vi "CD System Explorer lvlib.vi"(9 "Action":T1) -> (1 "Output":string)   [LabVIEW 2015, in "NIVS_Consolidated_CDW_MetaDataObj.lvclass"]
doc: "Constants, which are necessary for the <B>CD System Explorer library</B> in the generated custom device project."
uses:
  NIVS_Consolidated_CDW_MetaDataObj.lvclass
  CD System Explorer lvlib.ctl
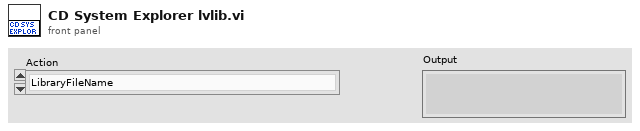
[diagram p1: front panel]
types:
  T1 = typedef "NIVS_Consolidated_CDW_MetaDataObj.lvclass/CD System Explorer lvlib.ctl" = enum16{"LibraryFileName", "LibraryFolderName", "System Explorer.FolderName", "System Explorer.Dynamically Called.FolderName", "System Explorer.Dynamically Called.Extra Pages.FolderName", "System Explorer.Dynamically Called.Extra Pages.TemplatePathAndName", "System Explorer.Dynamically Called.Main Page.VIName", "System Explorer.Dynamically Called.Main Page.TemplatePathAndName", "System Explorer.Dynamically Called.Initialization VI.VIName", "System Explorer.Dynamically Called.Initialization VI.TemplatePathAndName", "System Explorer.SubVI.FolderName", "System Explorer.Types.FolderName", "System Explorer.ActionVIOnCompile.VIName", "System Explorer.ExportConfigRTM.VIName", "System Explorer.LoadHelpFile.VIName"}
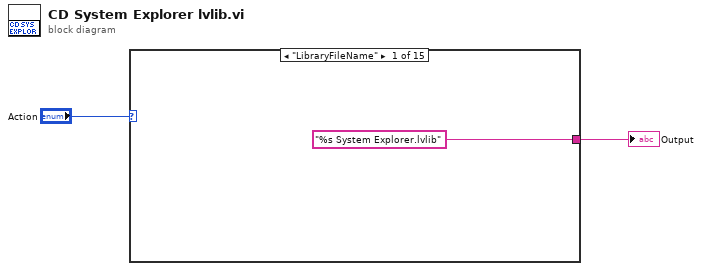
[diagram p0: block diagram]
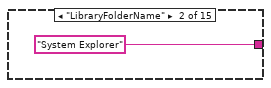
[diagram p2: hidden frame]
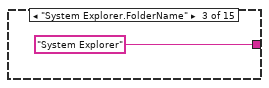
[diagram p3: hidden frame]
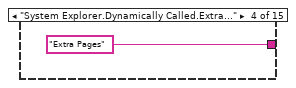
[diagram p4: hidden frame]
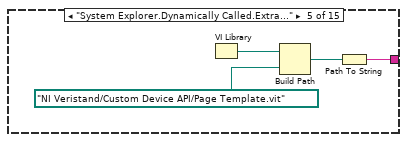
[diagram p5: hidden frame]
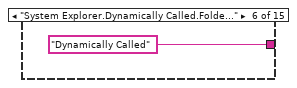
[diagram p6: hidden frame]
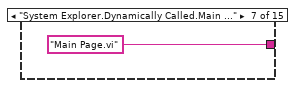
[diagram p7: hidden frame]
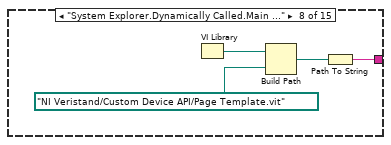
[diagram p8: hidden frame]
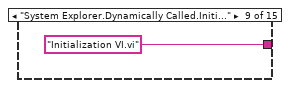
[diagram p9: hidden frame]
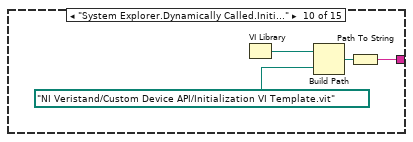
[diagram p10: hidden frame]
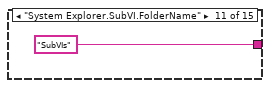
[diagram p11: hidden frame]
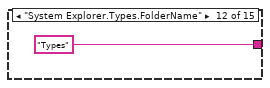
[diagram p12: hidden frame]
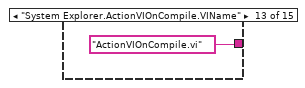
[diagram p13: hidden frame]
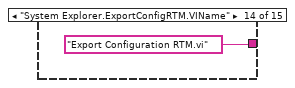
[diagram p14: hidden frame]
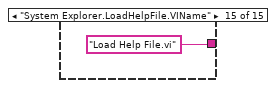
[diagram p15: hidden frame]
diagram:
  n1 = case shown="\"LibraryFileName\"" "Action" {
    tunnel: ["%s System Explorer.lvlib" "System Explorer" "System Explorer" "Extra Pages" w7 "Dynamically Called" "Main Page.vi" w14 "Initialization VI.vi" w18 "SubVIs" "Types" "ActionVIOnCompile.vi" ("name or relative path") "Export Configuration RTM.vi" ("Output") "Load Help File.vi" ("Output")] -> w2
    frame "LibraryFileName" {
    }
    frame "LibraryFolderName" {
    }
    frame "System Explorer.FolderName" {
    }
    frame "System Explorer.Dynamically Called.Extra Pages.FolderName" {
    }
    frame "System Explorer.Dynamically Called.Extra Pages.TemplatePathAndName" {
      n2 = VI Library() -> (path=w10:path)
      n3 = Build Path(base path=w10, name or relative path=path "NI Veristand/Custom Device API/Page Template.vit") -> (appended path=w8:path)
      n4 = Path To String(path=w8) -> (string=w7:string)
    }
    frame "System Explorer.Dynamically Called.FolderName" {
    }
    frame "System Explorer.Dynamically Called.Main Page.VIName" {
    }
    frame "System Explorer.Dynamically Called.Main Page.TemplatePathAndName" {
      n5 = VI Library() -> (path=w16:path)
      n6 = Build Path(base path=w16, name or relative path=path "NI Veristand/Custom Device API/Page Template.vit") -> (appended path=w13:path)
      n7 = Path To String(path=w13) -> (string=w14:string)
    }
    frame "System Explorer.Dynamically Called.Initialization VI.VIName" {
    }
    frame "System Explorer.Dynamically Called.Initialization VI.TemplatePathAndName" {
      n8 = VI Library() -> (path=w21:path)
      n9 = Build Path(base path=w21, name or relative path=path "NI Veristand/Custom Device API/Initialization VI Template.vit") -> (appended path=w19:path)
      n10 = Path To String(path=w19) -> (string=w18:string)
    }
    frame "System Explorer.SubVI.FolderName" {
    }
    frame "System Explorer.Types.FolderName" {
    }
    frame "System Explorer.ActionVIOnCompile.VIName" {
    }
    frame "System Explorer.ExportConfigRTM.VIName" {
    }
    frame "System Explorer.LoadHelpFile.VIName" {
    }
  }
  "Output" <- w2
